vi "Read_Instr.vi"(8 "error in (no error)":errorcluster caption="entrée d'erreur (pas d'erreur)", 11 "Class Instrument Patterm_Matching en entrée":refnum<class "Class Instrument Patterm_Matching.lvclass">) -> (0 "error out":errorcluster caption="sortie d'erreur", 3 "Class Instrument Patterm_Matching en sortie":refnum<class "Class Instrument Patterm_Matching.lvclass">)   [LabVIEW 2020, in "Library Instrument & Equipement.lvlib" / "Library Instruments.lvlib" / "Class Instrument Patterm_Matching.lvclass"]
uses:
  Class Instrument Patterm_Matching.lvclass
  Class Instrument Patterm_Matching.lvclass/Class Instrument Patterm_Matching.ctl
  Instrument (Default)/Class Instrument (Default).lvclass
  Camera/Class Camera Pattern Matching (Default)/Class Pattern Matching (Default).lvclass
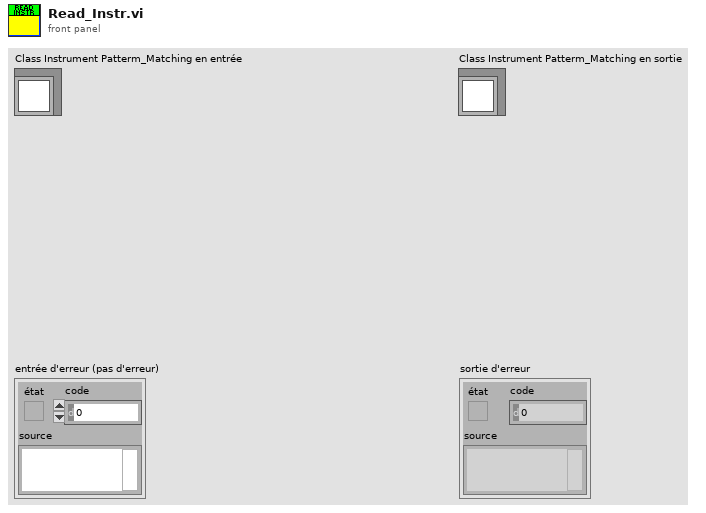
[diagram p1: front panel]
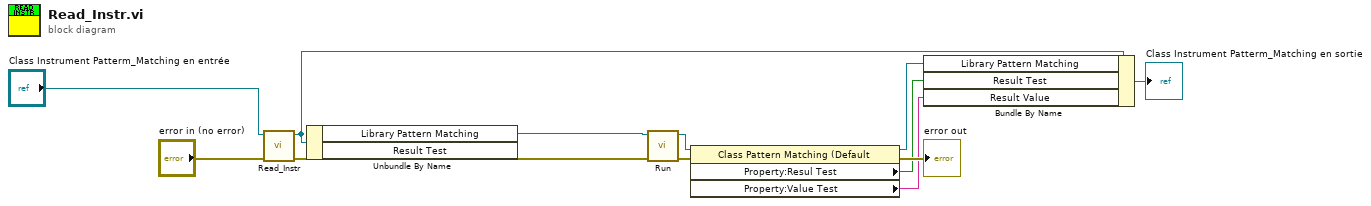
[diagram p0: block diagram]
diagram:
  n1 = call-parent "Read_Instr.vi"("error in (no error)"="error in (no error)", "Class Instrument (Default) en entrée"="Class Instrument Patterm_Matching en entrée") -> ("error out"=w10:errorcluster, "Class Instrument (Default) en sortie"=w9:refnum<class "Class Instrument Patterm_Matching.lvclass">)  [unwired: 8 in]
  n2 = Unbundle By Name(w9) -> ("Library Pattern Matching"=w1:refnum<class "Class Pattern Matching (Default).lvclass">)  [unwired: 1 out]
  n3 = call-dynamic "Run.vi"("error in (no error)"=w10, "Class Camera IV3-500CA en entrée"=w1) -> ("error out"=w7:errorcluster, "Class Camera IV3-500CA en sortie"=w6:refnum<class "Class Pattern Matching (Default).lvclass">)  [unwired: 8 in]
  n4 = property class="Class Pattern Matching (Default"(reference=w6, error in=w7) -> (reference out=w5:refnum<class "Class Pattern Matching (Default).lvclass">, error out=→"error out":errorcluster, "Property:Resul Test "=w3:bool, "Property:Value Test"=w2:string)
  n5 = Bundle By Name(cluster=w9, "Library Pattern Matching"=w5, "Result Test"=w3, "Result Value"=w2) -> (→"Class Instrument Patterm_Matching en sortie":refnum<class "Class Instrument Patterm_Matching.lvclass">)
